vi "err check.vi"(8 "error in (no error)":errorcluster, 11 "Acopian in":refnum<class "Acopian.lvclass">) -> (0 "error out":errorcluster, 3 "Acopian out":refnum<class "Acopian.lvclass">)   [LabVIEW 2019, in "Acopian.lvlib" / "Acopian.lvclass"]
uses:
  Library/Acopian.lvclass
  Library/Acopian.lvclass/Acopian.ctl
  Accessors/Read Local Resource.vi
  Accessors/Write Local Resource.vi
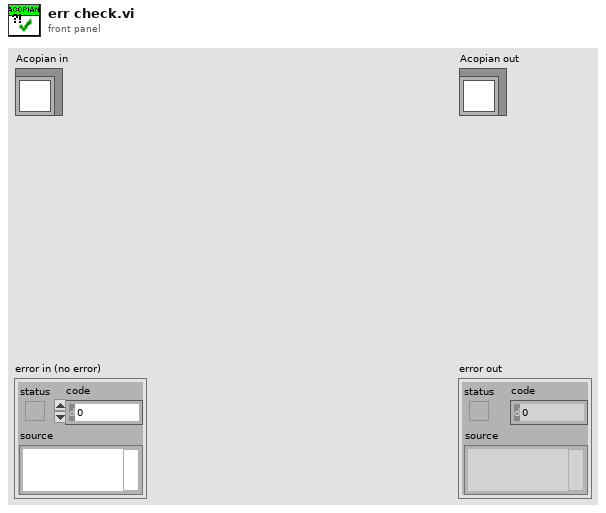
[diagram p1: front panel]
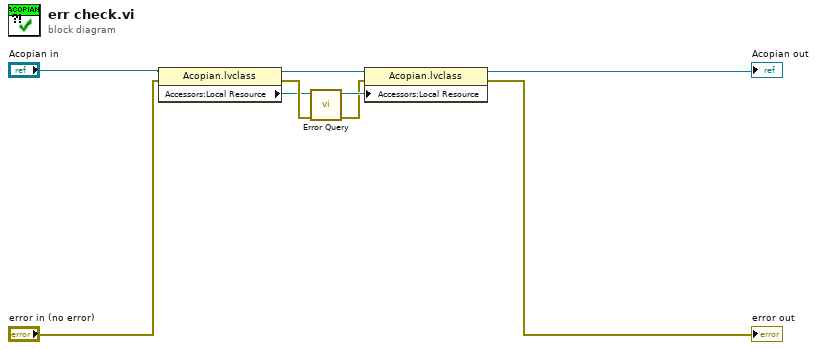
[diagram p0: block diagram]
diagram:
  n1 = property class="Acopian.lvclass"(reference="Acopian in", error in="error in (no error)") -> (reference out=w7:refnum<class "Acopian.lvclass">, error out=w6:errorcluster, "Accessors:Local Resource"=w5:refnum<visa-resource-name>)
  n2 = call "Error Query.vi"("error in"=w6, "VISA resource in"=w5) -> ("error out"=w8:errorcluster, "VISA resource out"=w9:refnum<visa-resource-name>)  [unwired: 6 in, 2 out]
  n3 = property class="Acopian.lvclass"(reference=w7, error in=w8, "Accessors:Local Resource"=w9) -> (reference out=→"Acopian out":refnum<class "Acopian.lvclass">, error out=→"error out":errorcluster)
